vi "Flatten.vi"(4 "T_Out":u64, 6 "T0":u64, 8 "error in (no error)":errorcluster, 10 "Data in":T1[](array[typedef]) {"Tags" format="%.0x"; "payload" format="%x"; "identifier" format="%x"}, 11 "CIFTag in":refnum<class "CIF_NIChn_FifoCAN.lvclass">) -> (0 "error out":errorcluster, 3 "CIFTag out":refnum<class "CIF_NIChn_FifoCAN.lvclass">)   [LabVIEW 2021, in "CIF_NIChn_FifoCAN.lvclass"]
uses:
  CIF_NIChn_FifoCAN.lvclass
  D:/dev/CIF-LVCore/src/Channels/CIFChannels/CIFChannels.lvclass
  ChannelCommon/typedef/Datatype CAN.ctl
  CIFChannels/CIFChannels.lvclass/CIFChannels.ctl
  CIF_NIChn_FifoCAN.lvclass/CIF_NIChn_FifoCAN.ctl
  ChannelCommon/CIFFIFO/CIFfifo.lvclass/CIFfifo.ctl
  ChannelCommon/CIFFIFO/Accessors/Write T0.vi
  ChannelCommon/CIFFIFO/Accessors/Write T_Out.vi
  ChannelCommon/Utilities/Flatten Header.vi
  ChannelCommon/CIFFIFO/Flatten/CAN Flatten.vi/be899675-9489-4ae7-9bdb-bbc908cd9623.vi
  ChannelCommon/CIFFIFO/Flatten/CAN Flatten.vi/fa4e04b0-1c28-4039-87e0-9391600efeb5.vi
  ChannelCommon/CIFFIFO/Flatten/CAN Flatten.vi/24dfac9c-4f7b-471b-adb6-3e40fb284e05.vi
  ChannelCommon/CIFFIFO/Accessors/Write Payload Length.vi
  ChannelCommon/CIFFIFO/Accessors/Read Header.vi
  CIFCore/Common/Utilities/Add Error.vi
  ChannelCommon/CIFFIFO/Flatten/CAN Flatten.vi/be899675-9489-4ae7-9bdb-bbc908cd9623.vi/c28b0ead-42ad-4072-80a2-aca7f2bd7ce3.vi
  ChannelCommon/CIFFIFO/Flatten/CAN Flatten.vi/fa4e04b0-1c28-4039-87e0-9391600efeb5.vi/c28b0ead-42ad-4072-80a2-aca7f2bd7ce3.vi
  ChannelCommon/CIFFIFO/Flatten/CAN Flatten.vi/24dfac9c-4f7b-471b-adb6-3e40fb284e05.vi/c28b0ead-42ad-4072-80a2-aca7f2bd7ce3.vi
  CIFCore/Common/Utilities/Append Error Location.vi
  ChannelCommon/Utilities/Update Time.vi
  ChannelCommon/CIFFIFO/CIFfifo.lvclass
  CIFChannels/CIFChannels.lvclass
  ChannelCommon/ChannelCommon.lvlib
panel:
  out "Data out":T1[](array[typedef]) {"Tags" format="%.0x"; "payload" format="%x"; "identifier" format="%x"}
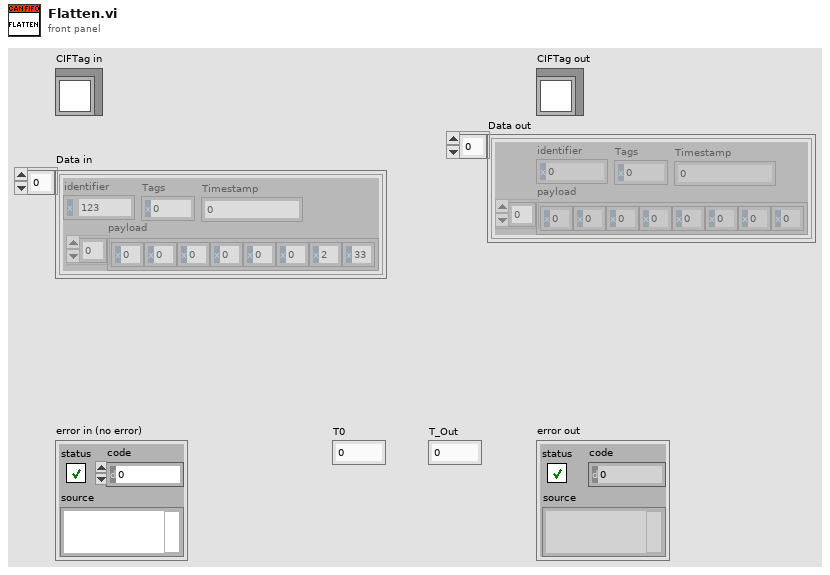
[diagram p1: front panel]
types:
  T1 = typedef "ChannelCommon.lvlib/Datatype CAN.ctl" = cluster{"payload":u8[], "identifier":u32, "Tags":u8, "Timestamp":u64}
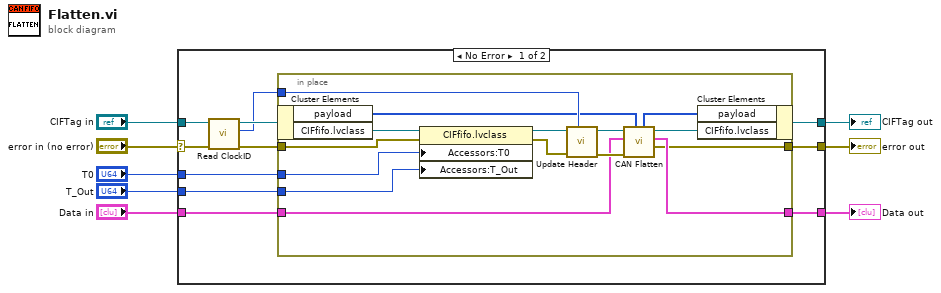
[diagram p0: block diagram]
diagram:
  n1 = case shown="No Error" "error in (no error)" {
    selector: "error in (no error)" -> [w12 w37]
    tunnel: [w17 w37] -> w7
    tunnel: [w16 w36] -> w5
    tunnel: "CIFTag in" -> [w15 w36]
    tunnel: "T_Out" -> [w19 _]
    tunnel: "T0" -> [w18 _]
    tunnel: "Data in" -> [w10 w35]
    tunnel: [w9 w35] -> w1
    frame No Error {
      n2 = call "Read ClockID.vi"("error in (no error)"=w12, "CIFChannels in"=w15) -> ("error out"=w11:errorcluster, "ClockID"=w13:u8, "CIFChannels out"=w14:refnum<class "CIF_NIChn_FifoCAN.lvclass">)  [unwired: 7 in]
      n3 = in-place {
        in-place-border: w19 -> [w31]
        in-place-border: w18 -> [w30]
        in-place-border: w11 -> [w29]
        in-place-border: [w20] -> w17
        in-place-border: w13 -> [w28]
        in-place-border: w10 -> [w25]
        in-place-border: [w24] -> w9
        n4 = in-place-cluster #1(w14) -> ("payload"=w23:u8[], "CIFfifo.lvclass"=w34:refnum<class "CIFfifo.lvclass">)
        n5 = property class="CIFfifo.lvclass"(reference=w34, error in=w29, "Accessors:T0"=w30, "Accessors:T_Out"=w31) -> (reference out=w33:refnum<class "CIFfifo.lvclass">, error out=w32:errorcluster)
        n6 = call "Update Header.vi"("ClockID"=w28, "error in (no error)"=w32, "CIFFIFO in"=w33) -> ("error out"=w26:errorcluster, "CIFFIFO out"=w27:refnum<class "CIFfifo.lvclass">)  [unwired: 7 in]
        n7 = call "CAN Flatten.vi"("payload in"=w23, "error in (no error)"=w26, "Data in"=w25, "CIFFifo in"=w27) -> ("error out"=w20:errorcluster, "Data out"=w24:T1[], "CIFFifo out"=w21:refnum<class "CIFfifo.lvclass">, "payload out"=w22:u8[])  [unwired: 4 in]
        n8 = in-place-cluster #1("payload"=w22, "CIFfifo.lvclass"=w21) -> (w16:refnum<class "CIF_NIChn_FifoCAN.lvclass">)
      }
    }
    frame Error {
    }
  }
  "error out" <- w7
  "CIFTag out" <- w5
  "Data out" <- w1
